vi "rd_readFile.vi"(6 "length":u64, 8 "error in (no error)":errorcluster, 9 "start index":u64, 10 "channel index":u32, 11 "Excel refumn":T3) -> (0 "error out":errorcluster, 3 "data_AllTypeData":T1)   [LabVIEW 2017, in "NI_ExcelFile.lvlib"]
uses:
  <vilib>/express/express shared/NI_ExcelFile/NI_ExcelFile.lvlib
  <vilib>/express/express shared/NI_ExcelFile/Ctrls/ExcelRefnum.ctl
  <vilib>/express/express shared/NI_ExcelFile/Ctrls/MainData.ctl
  <vilib>/express/express shared/NI_ExcelFile/Ctrls/StreamMode.ctl
  <vilib>/express/express shared/NI_ExcelFile/Ctrls/TimeColumnMode.ctl
  <vilib>/express/express shared/NI_ExcelFile/Ctrls/FileAttribute.ctl
  <vilib>/express/express shared/NI_ExcelFile/Ctrls/Columns.ctl
  <vilib>/express/express shared/NI_ExcelFile/Ctrls/ColumnInfo.ctl
  <vilib>/express/express shared/NI_ExcelFile/Ctrls/DataType.ctl
  <vilib>/express/express shared/NI_ExcelFile/Ctrls/wd_recordInfo.ctl
  <vilib>/express/express shared/NI_ExcelFile/Ctrls/disk_TemplateFile.ctl
  <vilib>/express/express shared/NI_ExcelFile/Ctrls/meta_file.ctl
  <vilib>/express/express shared/NI_ExcelFile/Ctrls/meta_Block.ctl
  <vilib>/express/express shared/NI_ExcelFile/Ctrls/meta_BlockType.ctl
  <vilib>/express/express shared/NI_ExcelFile/Ctrls/data_AllTypeData.ctl
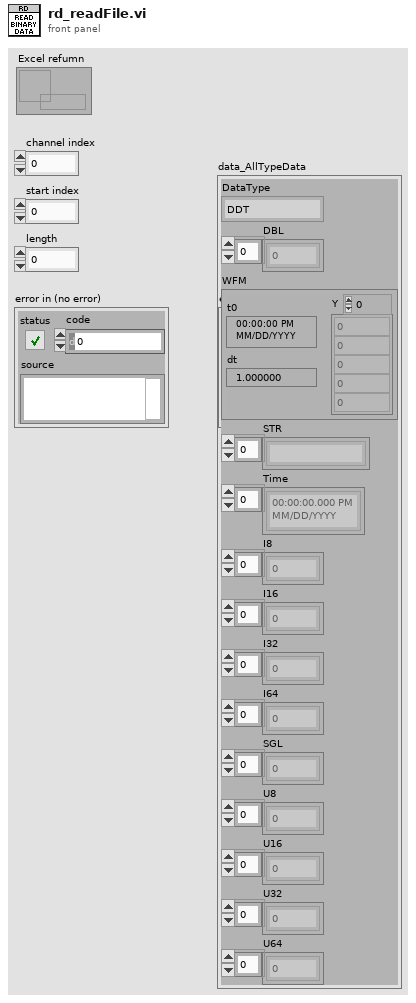
[diagram p1: front panel]
types:
  T1 = typedef "NI_ExcelFile.lvlib/data_AllTypeData.ctl" = cluster{"DataType":T2, "DBL":dbl[], "WFM":waveform(dbl), "STR":string[], "Time":timestamp[], "I8":i8[], "I16":i16[], "I32":i32[], "I64":i64[], "SGL":sgl[], "U8":u8[], "U16":u16[], "U32":u32[], "U64":u64[]}
  T2 = typedef "NI_ExcelFile.lvlib/DataType.ctl" = enum16{"DDT", "WFM", "Array of STR", "Array of DBL", "Array of I8", "Array of I16", "Array of I32", "Array of I64", "Array of SGL", "Array of U8", "Array of U16", "Array of U32", "Array of U64", "Array of Time"}
  T3 = typedef "NI_ExcelFile.lvlib/ExcelRefnum.ctl" = refnum<data-value>
  T4 = typedef "NI_ExcelFile.lvlib/MainData.ctl" = cluster{"TargetFile":path, "StreamMode":T5, "Append?":bool, "ChunkSize":u64, "TimeColumnMode":T6, "TimestampFormat":string, "AbsoluteTime?":bool, "FileAttribute ":T7, "Column":T8, "FileRef":refnum<k1>, "MemoryRef":refnum<data-value>[], "RecordInfo":T10[], " ChannelPreviousInfo":u32[], "ChannelFirstRecord":u32[], "PredefinedFormattedValueLength":i64, "DiskTemplate":T11}
  T5 = typedef "NI_ExcelFile.lvlib/StreamMode.ctl" = enum16{"File", "Memory"}
  T6 = typedef "NI_ExcelFile.lvlib/TimeColumnMode.ctl" = enum16{"Empty", "OnePerCh", "One"}
  T7 = typedef "NI_ExcelFile.lvlib/FileAttribute.ctl" = cluster{"Creator":string, "Title":string, "SheetName":string}
  T8 = typedef "NI_ExcelFile.lvlib/Columns.ctl" = T9[]
  T9 = typedef "NI_ExcelFile.lvlib/ColumnInfo.ctl" = cluster{"Header":string, "Format":string, "DataType":T2, "Length":u64}
  T10 = typedef "NI_ExcelFile.lvlib/wd_recordInfo.ctl" = cluster{"ChannelIndex":u32, "StartIndex":u64, "Length":u64, "Previous":i32, "Next":i32}
  T11 = typedef "NI_ExcelFile.lvlib/disk_TemplateFile.ctl" = cluster{"XMLRef":refnum<file>[], "ZipPath":path, "MetaFile":T12, "TempFolder":path}
  T12 = typedef "NI_ExcelFile.lvlib/meta_file.ctl" = cluster{"Ref":refnum<file>, "NextRow":i32, "NextPosition":i64, "Block":T13[]}
  T13 = typedef "NI_ExcelFile.lvlib/meta_Block.ctl" = cluster{"Version":u16, "Type":T14, "Length":i32, "Data":string}
  T14 = typedef "NI_ExcelFile.lvlib/meta_BlockType.ctl" = enum16{"NITag", "File", "Column"}
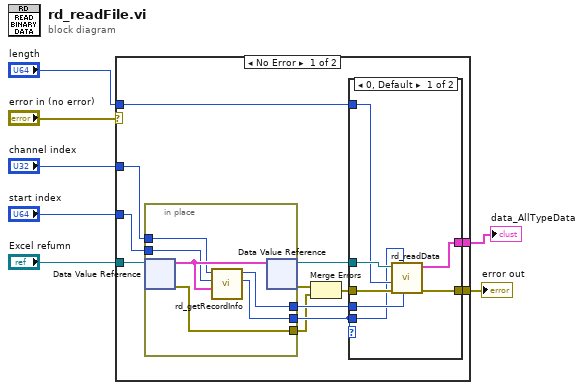
[diagram p0: block diagram]
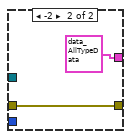
[diagram p2: hidden frame]
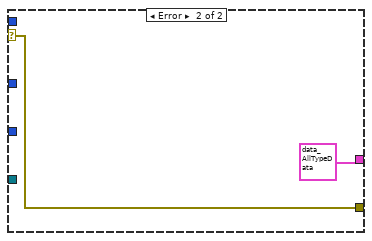
[diagram p3: hidden frame]
diagram:
  n1 = case shown="No Error" "error in (no error)" {
    selector: "error in (no error)" -> [_ w36]
    tunnel: "Excel refumn" -> [w19 _]
    tunnel: "channel index" -> [w18 _]
    tunnel: "start index" -> [w17 _]
    tunnel: [w14 T1 {"DataType"=enum."DDT", "DBL"=[], "WFM"={"t0"=timestamp(0 s since 1904-01-01), "dt"=1.0, "Y"=[]}, "STR"=[], "Time"=[], "I8"=[], "I16"=[], "I32"=[], "I64"=[], "SGL"=[], "U8"=[], "U16"=[], "U32"=[], "U64"=[]} ("fmt_AllTypeData")] -> w1
    tunnel: [w13 w36] -> w4
    tunnel: "length" -> [w11 _]
    frame No Error {
      n2 = in-place {
        in-place-border: [w33] -> w15
        in-place-border: [w30] -> w12
        in-place-border: w18 -> [w32]
        in-place-border: w17 -> [w31]
        in-place-border: [w29] -> w8
        n3 = in-place-dvr #1(w19) -> (w34:T4, w29:errorcluster)
        n4 = call <vilib>:"rd_getRecordInfo.vi"("meta in"=w34, "start index"=w31, "channel index"=w32) -> ("record index"=w30:i32, "record start index"=w33:u64)  [unwired: 7 in]
        n5 = in-place-dvr #1(w34) -> (w10:T3, w16:errorcluster)
      }
      n6 = Merge Errors(w16, w8) -> (w9:errorcluster)
      n7 = case shown="0, Default" w12 {
        tunnel: w10 -> [w26 _]
        tunnel: w11 -> [w25 _]
        tunnel: w9 -> [w24 w28]
        tunnel: w15 -> [w23 _]
        tunnel: w12 -> [w22 _]
        tunnel: [w20 T1 {"DataType"=enum."DDT", "DBL"=[], "WFM"={"t0"=timestamp(0 s since 1904-01-01), "dt"=1.0, "Y"=[]}, "STR"=[], "Time"=[], "I8"=[], "I16"=[], "I32"=[], "I64"=[], "SGL"=[], "U8"=[], "U16"=[], "U32"=[], "U64"=[]} ("fmt_AllTypeData")] -> w14
        tunnel: [w21 w28] -> w13
        frame 0, Default {
          n8 = call <vilib>:"rd_readData.vi"("record start"=w23, "record index"=w22, "error in (no error)"=w24, "length"=w25, "Excel refnum"=w26) -> ("error out"=w21:errorcluster, "data_AllTypeData"=w20:T1)  [unwired: 4 in, 1 out]
        }
        frame -2 {
        }
      }
    }
    frame Error {
    }
  }
  "error out" <- w4
  "data_AllTypeData" <- w1
